vi "Release.vi"(8 "error in (no error)":errorcluster, 11 "PropertyObject in":refnum<class "PropertyObject.lvclass">) -> (0 "error out":errorcluster)   [LabVIEW 2020, in "TSnax.lvlib" / "PropertyObject.lvclass"]
uses:
  PropertyObject.lvclass
  PropertyObject.lvclass/PropertyObject.ctl
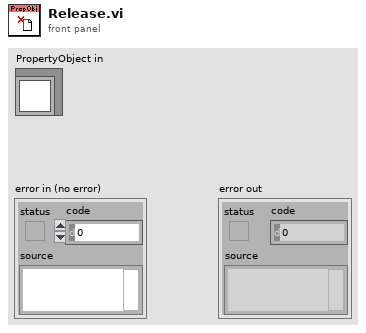
[diagram p1: front panel]
types:
  T1 = typedef "TSnax.lvlib/PropertyObject.lvclass/Ref Data.ctl" = cluster{"PropertyObject":refnum<k7>}
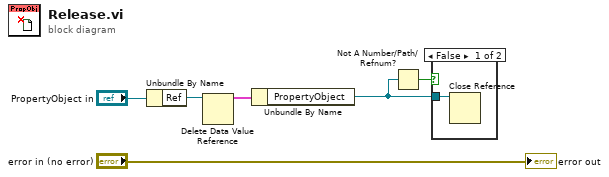
[diagram p0: block diagram]
diagram:
  n1 = Unbundle By Name("PropertyObject in") -> ("Ref"=w2:refnum<data-value>)
  n2 = Delete Data Value Reference(data value reference=w2) -> (data value=w1:T1)  [unwired: 1 in, 1 out]
  n3 = Unbundle By Name(w1) -> ("PropertyObject"=w5:refnum<k7>)
  n4 = Not A Number/Path/Refnum?(number/path/refnum=w5) -> (NaN/Path/Refnum?=w4:bool)
  n5 = case shown="False" w4 {
    tunnel: w5 -> [w7 _]
    frame False {
      n6 = Close Reference(reference=w7) -> ()  [unwired: 1 in, 1 out]
    }
    frame True {
    }
  }
  "error out" <- "error in (no error)"
